vi "Execution_Event_SendDataToMessageHandler.vi"(8 "error in (no error)":errorcluster, 10 "Message":refnum<class "Messages.lvclass">, 11 "EVE in":refnum<class "EVE.lvclass">) -> (0 "error out":errorcluster, 3 "EVE out":refnum<class "EVE.lvclass">)   [LabVIEW 2013, in "EVE.lvclass"]
uses:
  EVE.lvclass
  Messages/Messages.lvclass
  EVE.lvclass/EVE.ctl
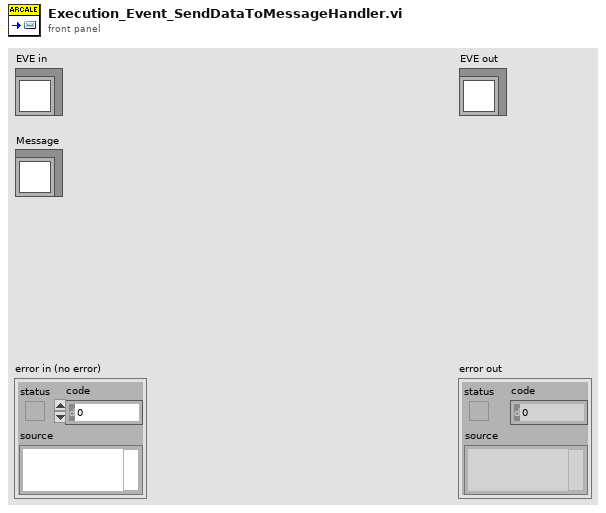
[diagram p1: front panel]
types:
  T1 = typedef "usereventprio.ctl" = enum32{"high priority", "normal priority"}
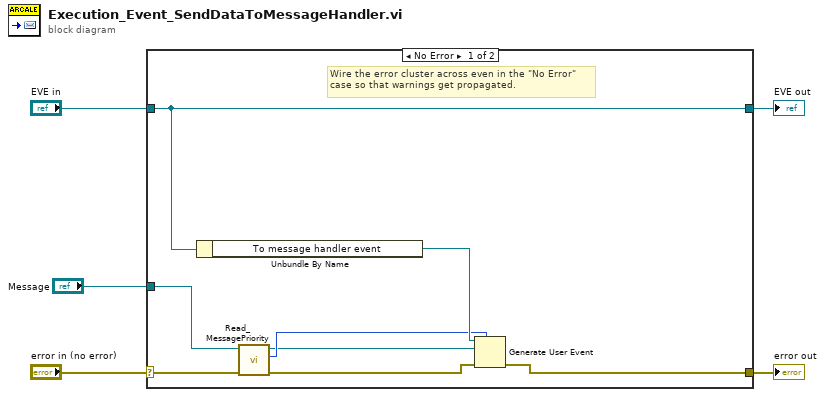
[diagram p0: block diagram]
diagram:
  n1 = case shown="No Error" "error in (no error)" {
    selector: "error in (no error)" -> [w9 w15]
    tunnel: [w11 w15] -> w4
    tunnel: [w13 w14] -> w2
    tunnel: "EVE in" -> [w13 w14]
    tunnel: "Message" -> [w10 _]
    frame No Error {
      # "Wire the error cluster across even in the \"No Error\"\ncase so that warnings get propagated."
      n2 = Unbundle By Name(w13) -> ("To message handler event"=w12:refnum<user-event>)
      n3 = call-dynamic "Read_MessagePriority.vi"("error in (no error)"=w9, "Messages in"=w10) -> ("error out"=w8:errorcluster, "user event priority"=w7:T1, "Messages out"=w6:refnum<class "Messages.lvclass">)  [unwired: 7 in]
      n4 = Generate User Event(priority (normal)=w7, user event=w12, event data cluster=w6, error in=w8) -> (error out=w11:errorcluster)  [unwired: 1 out]
    }
    frame Error {
    }
  }
  "error out" <- w4
  "EVE out" <- w2
